vi "GenCodeScripts-AddSubVI.vi"(8 "error in (no error)":errorcluster, 9 "path":path, 10 "Terms":T2, 11 "Diagram":T1) -> (0 "error out":errorcluster, 2 "Terms (dup)":T2, 3 "Diagram (dup)":T1)   [LabVIEW 2014, in "TagDB(dev).lvlib"]
uses:
  TagDB(dev).lvlib
  <vilib>/XNodeSupport/XNodeTopLevelDiagramRef.ctl
  <vilib>/XNodeSupport/XNodeTermIDPairs.ctl
  <vilib>/XNodeSupport/XNodeTermIDPair.ctl
  <vilib>/XNodeSupport/XNodeTermRef.ctl
  <vilib>/XNodeSupport/XNodeString.ctl
  <vilib>/XNodeSupport/NI_XNodeSupport.lvlib
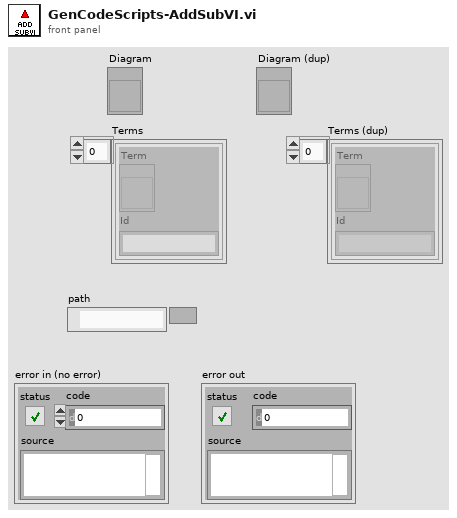
[diagram p1: front panel]
types:
  T1 = typedef "NI_XNodeSupport.lvlib/XNodeTopLevelDiagramRef.ctl" = refnum<vi>
  T2 = typedef "NI_XNodeSupport.lvlib/XNodeTermIDPairs.ctl" = T3[]
  T3 = typedef "NI_XNodeSupport.lvlib/XNodeTermIDPair.ctl" = cluster{"Term":T4, "Id":T5}
  T4 = typedef "NI_XNodeSupport.lvlib/XNodeTermRef.ctl" = refnum<vi>
  T5 = typedef "NI_XNodeSupport.lvlib/XNodeString.ctl" = string
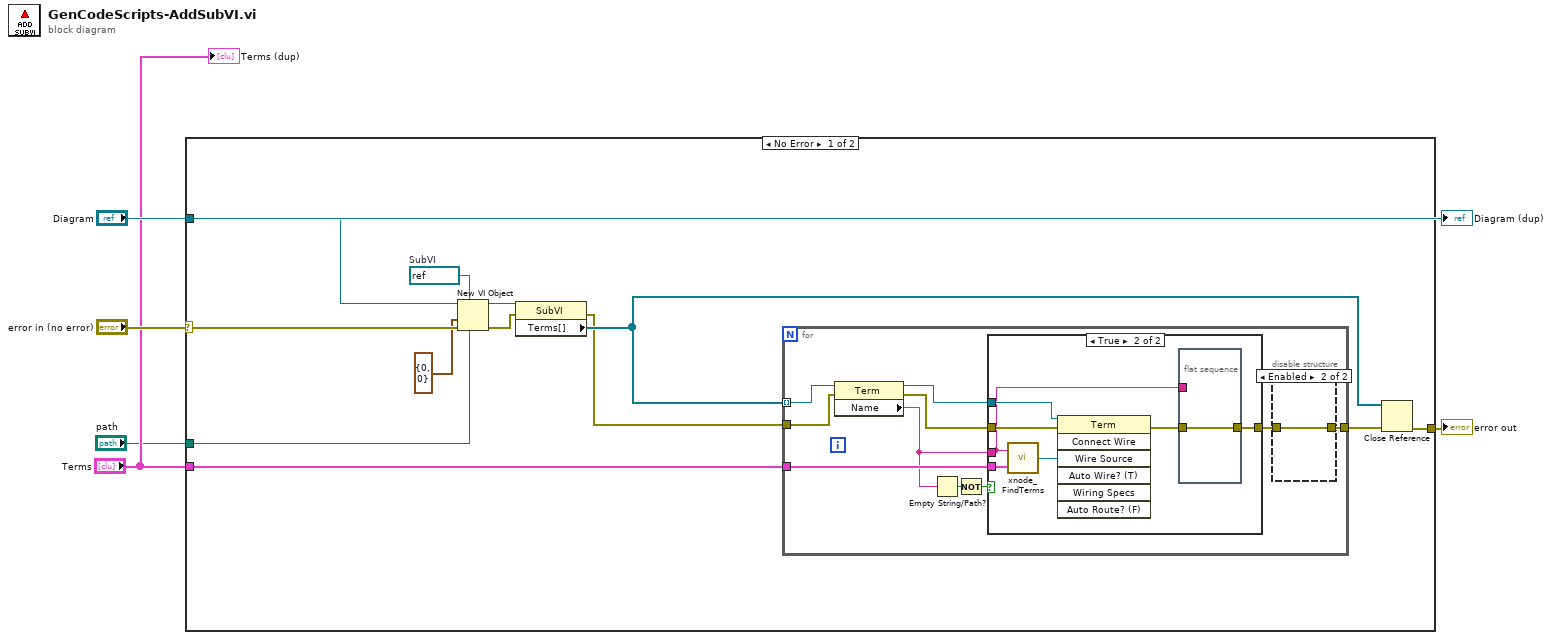
[diagram p0: block diagram]
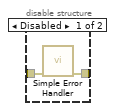
[diagram p2: hidden frame]
diagram:
  n1 = case shown="No Error" "error in (no error)" {
    selector: "error in (no error)" -> [w17 w40]
    tunnel: [w16 w40] -> w4
    tunnel: "Diagram" -> [w8 _]
    tunnel: "Terms" -> [w7 _]
    tunnel: "path" -> [w6 _]
    frame No Error {
      w10 = refnum<vi> refnum  # SubVI
      n2 = New VI Object(vi object class=w10, owner refnum=w8, position/next to=cluster{"Horizontal":i16, "Vertical":i16} {"Horizontal"=0, "Vertical"=0}, 6:w6, 8:w17) -> (object refnum=w11:refnum<vi>, 0:w15:errorcluster)  [unwired: 3 in]
      n3 = property class="SubVI"(reference=w11, error in=w15) -> (error out=w13:errorcluster, "Terms[]"=w14:refnum<vi>[])  [unwired: 1 out]
      n4 = for {
        tunnel: w7 -> [w27]
        tunnel: w14 -> [w26] mode=indexing
        tunnel: w13 -> [w24]
        tunnel: [w22] -> w12
        n5 = property class="Term"(reference=w26, error in=w24) -> (reference out=w25:refnum<vi>, error out=w23:errorcluster, "Name"=w20:string)
        n6 = Empty String/Path?(string/path=w20) -> (empty?=w19:bool)
        n7 = Not(x=w19) -> (.not. x?=w18:bool)
        n8 = case shown="True" w18 {
          tunnel: w27 -> [_ w38]
          tunnel: w25 -> [_ w36]
          tunnel: w23 -> [w31 w35]
          tunnel: w20 -> [_ w34]
          tunnel: [w31 w33] -> w21
          frame False {
          }
          frame True {
            n9 = call "xnode_FindTerms.vi"("Terms"=w38, "String"=w34) -> ("Terminal"=w37:T4)
            n10 = invoke class="Term" method="Connect Wire"(reference=w36, error in=w35, "Wire Source"=w37) -> (error out=w32:errorcluster)  [unwired: 4 in, 6 out]
            n11 = flat-sequence {
              tunnel: w34 -> [_]
              tunnel: [w39] -> w33
              tunnel: w32 -> [w39]
              frame #0 {
              }
            }
          }
        }
        n12 = disable-structure shown="Enabled" {
          disable-tunnel: [w29 w30] -> w22
          disable-tunnel: w21 -> [w28 w30]
          frame Disabled {
            n13 = call <vilib>:"Simple Error Handler.vi"("error in (no error)"=w28) -> ("error out"=w29:errorcluster)  [unwired: 4 in, 4 out]
          }
          frame Enabled {
          }
        }
      }
      n14 = Close Reference(reference=w14, error in (no error)=w12) -> (error out=w16:errorcluster)
    }
    frame Error {
    }
  }
  "error out" <- w4
  "Terms (dup)" <- "Terms"
  "Diagram (dup)" <- "Diagram"
